vi "Trimmer.vi"(8 "error in":errorcluster, 11 "String In":string) -> (0 "error out":errorcluster, 3 "result string":string)   [LabVIEW 2019]
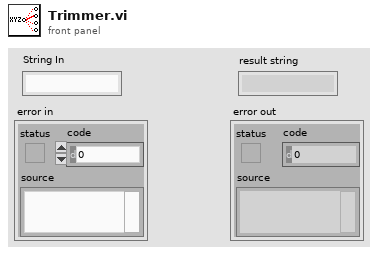
[diagram p1: front panel]
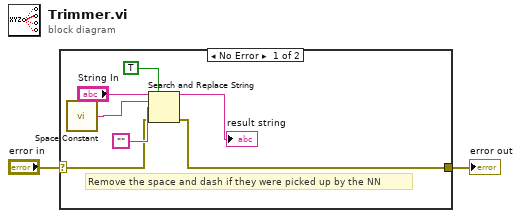
[diagram p0: block diagram]
diagram:
  n1 = case shown="No Error" "error in" {
    selector: "error in" -> [w6 w10]
    tunnel: [w5 w10] -> w1
    frame No Error {
      # "Remove the space and dash if they were picked up by the NN"
      n2 = call <vilib>:"Space Constant.vi"() -> ("String"=w8:string)
      n3 = Search and Replace String(replace all?=TRUE ("replace all? (F)"), input string="String In", search string=w8, replace string="", error in=w6) -> (result string=→"result string":string, error out=w5:errorcluster)  [unwired: 3 in, 2 out]
    }
    frame Error {
      # ":("
    }
  }
  "error out" <- w1
